vi "Clear Specific Error.vi"(8 "error in":errorcluster, 11 "Error Code":i32) -> (0 "error out":errorcluster)   [LabVIEW 2019, in "TSC Error.lvlib"]
doc: "This VI will clear a specific error code if that is the error on the wire.\n\nInputs:\n-Error Code [I32] - the error code to compare to and clear if it is the existing error\n-error in\n\nOutputs:\n-error out\n\n____________________________________\n<b>Code Developed By:</b>\nDaniel Coons\nTechnology Service Corporation\n1983 S Liberty Drive\nBloomington, IN 47403\nPhone: 812 558-7100\ndaniel.coons@tsc.com\nwww.tsc.com\n\n<b>Date Created:</b> 11 AUG 2014\n<b>Date Updated:</b>"
uses:
  TSC Error.lvlib
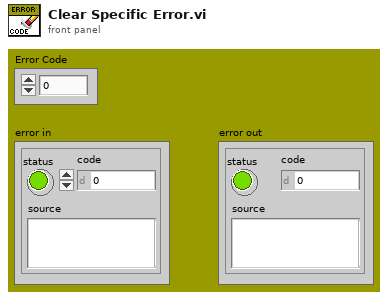
[diagram p1: front panel]
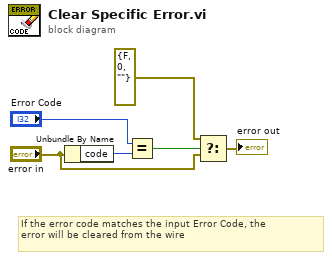
[diagram p0: block diagram]
diagram:
  # "If the error code matches the input Error Code, the \nerror will be cleared from the wire"
  n1 = Unbundle By Name("error in") -> ("code"=w3:i32)
  n2 = Equal?(x="Error Code", y=w3) -> (x = y?=w2:bool)
  n3 = Select(t=errorcluster {"status"=FALSE, "code"=0, "source"=""}, s=w2, f="error in") -> (s? t:f=→"error out":errorcluster)
